vi "Get gRPC ID.vi"(11 "OOP Server in":refnum<class "HVC6.lvclass">) -> (2 "gRPC ID":T1, 3 "OOP Server out":refnum<class "HVC6.lvclass">)   [LabVIEW 2019, in "HVC6.lvlib" / "HVC6.lvclass"]
uses:
  HVC6.lvclass
  gRPC lvSupport/Server API/typeDefs/grpcId.ctl
  HVC6.lvclass/HVC6.ctl
  gRPC lvSupport/gprc-lvsupport.lvlib
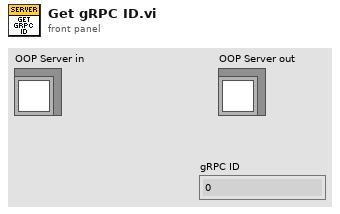
[diagram p1: front panel]
types:
  T1 = typedef "HVC6.lvlib/gprc-lvsupport.lvlib/grpcId.ctl" = u64
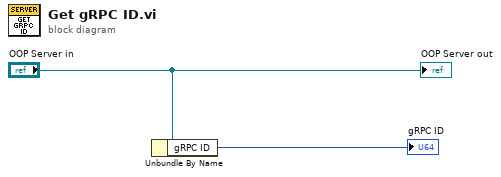
[diagram p0: block diagram]
diagram:
  n1 = Unbundle By Name("OOP Server in") -> ("gRPC ID"=→"gRPC ID":T1)
  "OOP Server out" <- "OOP Server in"
